vi "LC_Relay_Protection.vi"(0 "Protection settings":T4, 1 "Reset Relay":bool, 3 "RMS minimum\nvalues":cluster{"VRMS values":dbl, "IRMS values":dbl}, 5 "RMS values":dbl[](array[numeric]), 9 "Total power values":dbl[](array[numeric]), 11 "input cluster":T3, 12 "Blocking in":bool, 14 "Transfer Trip":bool) -> (4 "trip signal":bool, 6 "Reclose":bool, 8 "Relay State":cluster{"Lockout":bool, "State":i16}, 10 "Blocking out":bool[](array[boolean]), 13 "millisecond timer value":u32, 15 "output cluster":T3)   [LabVIEW 2016]
doc: "Compares voltage and current RMS values with user defined protection settings to detect undervoltage and overcurrent and calculate trip time.\nImplements definite time and inverse time protection."
uses:
  <vilib>/addons/Electrical Power/Protection/Definite Time Delay/subVIs/fpga_Timer Feedback Var.ctl
  <vilib>/addons/Electrical Power/Protection/Definite Time Delay/subVIs/fpga_State.ctl
  <vilib>/addons/Electrical Power/Protection/Inverse Time Delay/subVIs/ep_Operate Time.ctl
  <vilib>/addons/Electrical Power/Protection/NI_EP_Protection.lvlib
  <vilib>/addons/Electrical Power/Protection/NI_EP_Protection_FPGA.lvlib
panel:
  out "VL error":i32
  out "VR error":i32
  out "I error":i32
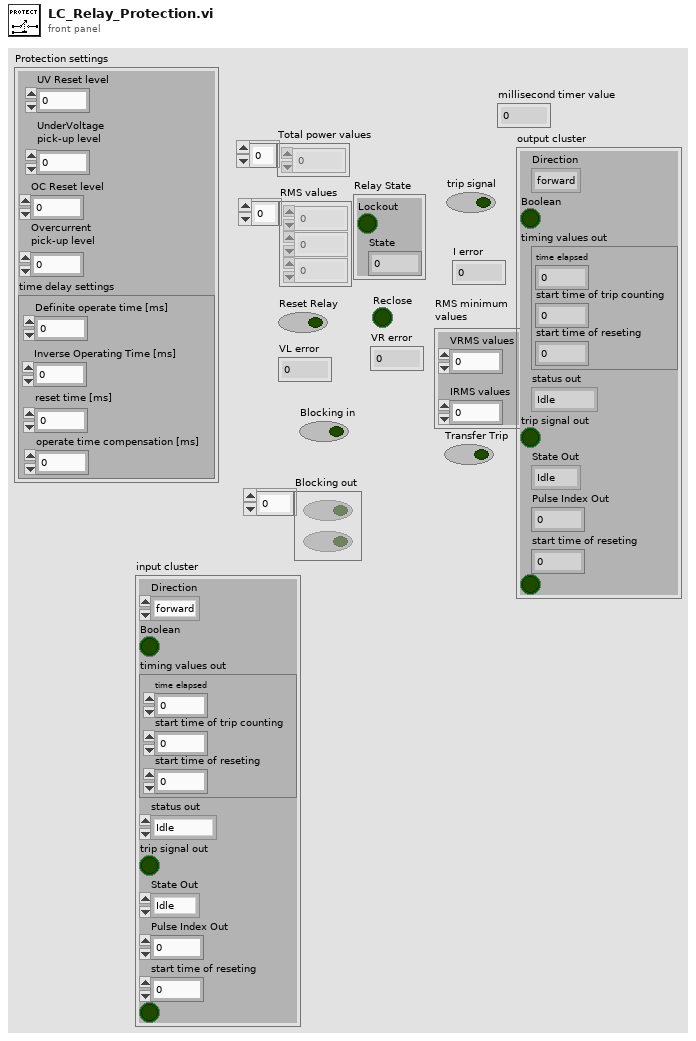
[diagram p1: front panel]
types:
  T1 = typedef "NI_EP_Protection_FPGA.lvlib/fpga_Timer Feedback Var.ctl" = cluster{"time elapsed":u32, "start time of trip counting":u32, "start time of reseting":u32}
  T2 = typedef "NI_EP_Protection_FPGA.lvlib/fpga_State.ctl" = enum16{"Idle", "Trip Counting", "Tripped", "Reset Counting"}
  T3 = cluster{"Direction":enum16{"forward", "backward", "N/D"}, "Boolean":bool, "timing values out":T1, "status out":T2, "trip signal out":bool, "State Out":enum16{"Idle", "Wait for Trip", "PulseClosing", "Locked"}, "Pulse Index Out":i32, "start time of reseting":u32, bool}
  T4 = cluster{"UV Reset level":dbl, "UnderVoltage \npick-up level":dbl, "OC Reset level":dbl, "Overcurrent\npick-up level":dbl, "time delay settings":cluster{"Definite operate time [ms]":u32, "Inverse Operating Time [ms]":u32, "reset time [ms]":u32, "operate time compensation [ms]":u32}}
  T5 = enum16{"Idle", "Wait for Trip", "PulseClosing", "Locked"}
  T6 = cluster{"Definite operate time [ms]":u32, "Inverse Operating Time [ms]":u32, "reset time [ms]":u32, "operate time compensation [ms]":u32}
  T7 = typedef "NI_EP_Protection.lvlib/ep_Operate Time.ctl" = cluster{"A [s]":dbl, "B [s]":dbl, "alpha":dbl, "K2 [s]":dbl, "K1 [s]":dbl, "K3 [s]":dbl}
  T8 = cluster{u32, "reset time [ms]":u32, "reset time [ms]":u32}
  T9 = cluster{"Definite operate time [ms]":u32, "reset time [ms]":u32, "reset time [ms]":u32}
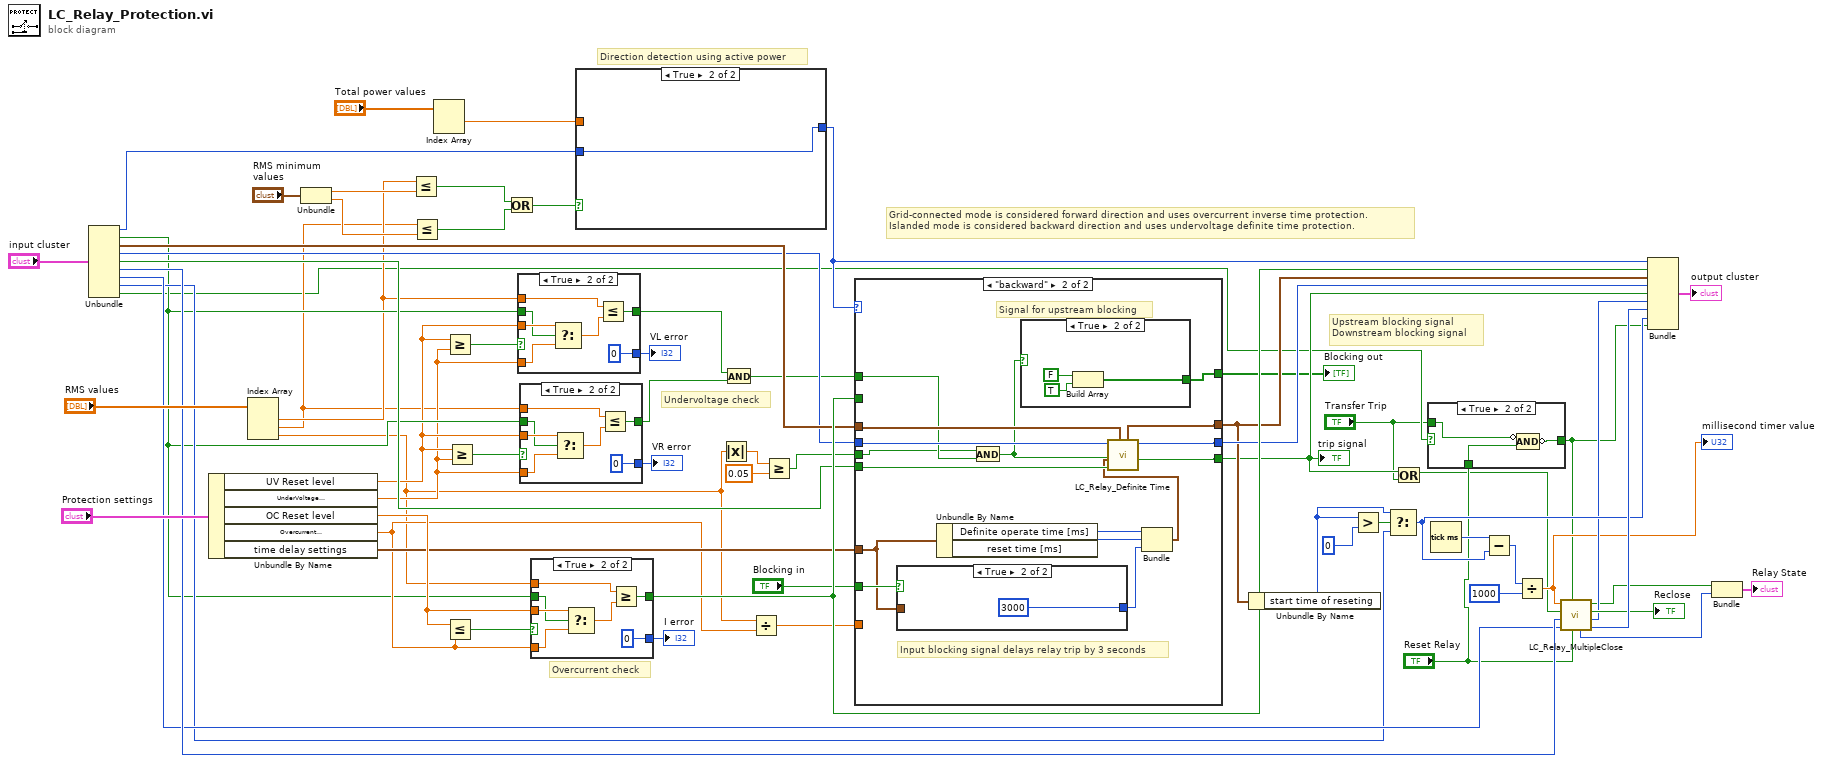
[diagram p0: block diagram]
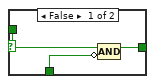
[diagram p2: hidden frame]
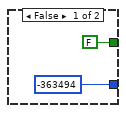
[diagram p3: hidden frame]
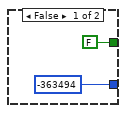
[diagram p4: hidden frame]
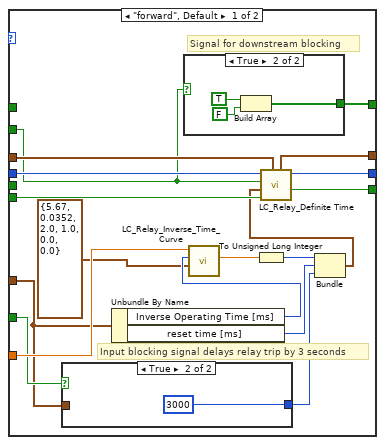
[diagram p5: hidden frame]
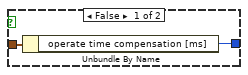
[diagram p6: hidden frame]
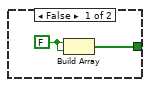
[diagram p7: hidden frame]
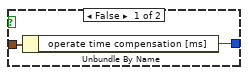
[diagram p8: hidden frame]
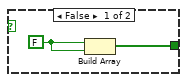
[diagram p9: hidden frame]
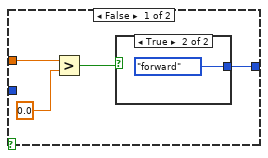
[diagram p10: hidden frame]
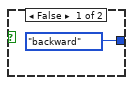
[diagram p11: hidden frame]
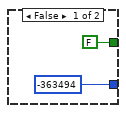
[diagram p12: hidden frame]
diagram:
  # "Grid-connected mode is considered forward direction and uses overcurrent inverse time protection.\nIslanded mode is considered backward direction and uses undervoltage definite time protection."
  # "Overcurrent check"
  # "Undervoltage check"
  # "Direction detection using active power"
  # "Upstream blocking signal\nDownstream blocking signal"
  n1 = Unbundle("input cluster") -> ("Direction"=w44:enum16{"forward", "backward", "N/D"}, "Boolean"=w25:bool, "timing values out"=w31:T1, "status out"=w30:T2, "trip signal out"=w29:bool, "State Out"=w28:T5, "Pulse Index Out"=w27:i32, "start time of reseting"=w26:u32, w7:bool)
  n2 = Unbundle By Name("Protection settings") -> ("UV Reset level"=w24:dbl, "UnderVoltage \npick-up level"=w23:dbl, "OC Reset level"=w59:dbl, "Overcurrent\npick-up level"=w46:dbl, "time delay settings"=w57:T6)
  n3 = Index Array(array="RMS values") -> (element #1=w22:dbl, element #2=w21:dbl, element #3=w18:dbl)  [unwired: 3 in]
  n4 = Unbundle("RMS minimum\nvalues") -> ("VRMS values"=w64:dbl, "IRMS values"=w61:dbl)
  n5 = Less Or Equal?(x=w22, y=w64) -> (x <= y?=w63:bool)
  n6 = Less Or Equal?(x=w21, y=w61) -> (x <= y?=w62:bool)
  n7 = Index Array(array="Total power values") -> (element #1=w50:dbl)  [unwired: 2 in, 1 out]
  n8 = Greater Or Equal?(x=w24, y=w23) -> (x >= y?=w33:bool)
  n9 = Less Or Equal?(x=w59, y=w46) -> (x <= y?=w67:bool)
  n10 = Greater Or Equal?(x=w24, y=w23) -> (x >= y?=w35:bool)
  n11 = Or(x=w63, y=w62) -> (x .or. y?=w54:bool)
  n12 = case shown="True" w33 {
    tunnel: [-363494 ("error") 0 ("error")] -> w32
    tunnel: w24 -> [_ w74]
    tunnel: w23 -> [_ w73]
    tunnel: [FALSE ("Boolean") w72] -> w20
    tunnel: w25 -> [_ w71]
    tunnel: w22 -> [_ w70]
    frame False {
    }
    frame True {
      n13 = Select(t=w74, s=w71, f=w73) -> (s? t:f=w76:dbl)
      n14 = Less Or Equal?(x=w70, y=w76) -> (x <= y?=w72:bool)
    }
  }
  "VL error" <- w32
  n15 = case shown="True" w35 {
    tunnel: [-363494 ("error") 0 ("error")] -> w34
    tunnel: w24 -> [_ w83]
    tunnel: w23 -> [_ w82]
    tunnel: [FALSE ("Boolean") w81] -> w19
    tunnel: w25 -> [_ w80]
    tunnel: w21 -> [_ w79]
    frame False {
    }
    frame True {
      n16 = Select(t=w83, s=w80, f=w82) -> (s? t:f=w85:dbl)
      n17 = Less Or Equal?(x=w79, y=w85) -> (x <= y?=w81:bool)
    }
  }
  "VR error" <- w34
  n18 = case shown="True" w67 {
    tunnel: [-363494 ("error") 0 ("error")] -> w66
    tunnel: w59 -> [_ w92]
    tunnel: w46 -> [_ w91]
    tunnel: [FALSE ("Boolean") w90] -> w58
    tunnel: w25 -> [_ w89]
    tunnel: w18 -> [_ w88]
    frame False {
    }
    frame True {
      n19 = Select(t=w92, s=w89, f=w91) -> (s? t:f=w94:dbl)
      n20 = Greater Or Equal?(x=w88, y=w94) -> (x >= y?=w90:bool)
    }
  }
  "I error" <- w66
  n21 = case shown="True" w54 {
    tunnel: w50 -> [w96 _]
    tunnel: w44 -> [_ w101]
    tunnel: [w95 w101] -> w43
    frame False {
      n22 = Greater?(x=w96, y=0.0) -> (0:w97:bool)
      n23 = case shown="True" w97 {
        tunnel: [enum16{"forward", "backward"}."backward" enum16{"forward", "backward"}."forward"] -> w95
        frame False {
        }
        frame True {
        }
      }
    }
    frame True {
    }
  }
  n24 = Absolute Value(x=w18) -> (abs(x)=w14:dbl)
  n25 = And(x=w20, y=w19) -> (x .and. y?=w16:bool)
  n26 = Divide(x=w18, y=w46) -> (x/y=w55:dbl)
  n27 = Greater Or Equal?(x=w14, y=0.05) -> (x >= y?=w15:bool)
  n28 = case shown="\"backward\"" w43 {
    tunnel: w58 -> [w102 _]
    tunnel: w57 -> [w105 w134]
    tunnel: [w119 w138] -> w56
    tunnel: w55 -> [w118 _]
    tunnel: [w117 w139] -> w53
    tunnel: [w103 w129] -> w47
    tunnel: w31 -> [w116 w142]
    tunnel: w30 -> [w115 w141]
    tunnel: w29 -> [w114 w140]
    tunnel: [w107 w137] -> w37
    tunnel: "Blocking in" -> [w106 w136]
    tunnel: w15 -> [_ w130]
    tunnel: w16 -> [_ w131]
    frame "forward", Default {
      # "Input blocking signal delays relay trip by 3 seconds"
      # "Signal for downstream blocking"
      n29 = case shown="True" w106 {
        tunnel: [w120 u32 3000 ("reset time [ms]")] -> w104
        tunnel: w105 -> [w121 _]
        frame False {
          n30 = Unbundle By Name(w121) -> ("operate time compensation [ms]"=w120:u32)
        }
        frame True {
        }
      }
      n31 = Unbundle By Name(w105) -> ("Inverse Operating Time [ms]"=w113:u32, "reset time [ms]"=w110:u32)
      n32 = case shown="True" w102 {
        tunnel: [w123 w125] -> w107
        frame False {
          w124 = FALSE
          n33 = Build Array(w124, w124) -> (w123:bool[])
        }
        frame True {
          n34 = Build Array(TRUE, FALSE) -> (w125:bool[])
        }
      }
      n35 = call "LC_Relay_Inverse_Time_Curve.vi"("input cluster"=T7 {"A [s]"=5.67, "B [s]"=0.0352, "alpha"=2.0, "K2 [s]"=1.0, "K1 [s]"=0.0, "K3 [s]"=0.0}, "time dial"=w113, "multiples of pickup"=w118) -> ("oparate time"=w111:dbl)  [unwired: 5 in, 1 out]
      n36 = To Unsigned Long Integer(number=w111) -> (unsigned 32bit integer=w108:u32)
      n37 = Bundle(w108, "reset time [ms]"=w110, "reset time [ms]"=w104) -> (w109:T8)  [unwired: 1 in]
      n38 = call "LC_Relay_Definite Time.vi"("timing values in"=w116, "trip signal in"=w114, "time delay settings"=w109, "pick-up signal? (F)"=w102, "status in"=w115) -> ("trip signal out"=w103:bool, "status out"=w119:T2, "timing values out"=w117:T1)  [unwired: 3 in, 1 out]
    }
    frame "backward" {
      # "Signal for upstream blocking"
      # "Input blocking signal delays relay trip by 3 seconds"
      n39 = case shown="True" w136 {
        tunnel: [w144 u32 3000 ("reset time [ms]")] -> w135
        tunnel: w134 -> [w145 _]
        frame False {
          n40 = Unbundle By Name(w145) -> ("operate time compensation [ms]"=w144:u32)
        }
        frame True {
        }
      }
      n41 = Unbundle By Name(w134) -> ("Definite operate time [ms]"=w133:u32, "reset time [ms]"=w143:u32)
      n42 = And(x=w130, y=w131) -> (x .and. y?=w128:bool)
      n43 = case shown="True" w128 {
        tunnel: [w147 w149] -> w137
        frame False {
          w148 = FALSE
          n44 = Build Array(w148, w148) -> (w147:bool[])
        }
        frame True {
          n45 = Build Array(FALSE, TRUE) -> (w149:bool[])
        }
      }
      n46 = Bundle("Definite operate time [ms]"=w133, "reset time [ms]"=w143, "reset time [ms]"=w135) -> (w132:T9)  [unwired: 1 in]
      n47 = call "LC_Relay_Definite Time.vi"("timing values in"=w142, "trip signal in"=w140, "time delay settings"=w132, "pick-up signal? (F)"=w128, "status in"=w141) -> ("trip signal out"=w129:bool, "status out"=w138:T2, "timing values out"=w139:T1)  [unwired: 3 in, 1 out]
    }
  }
  "trip signal" <- w47
  "Blocking out" <- w37
  n48 = Unbundle By Name(w53) -> ("start time of reseting"=w40:u32)
  n49 = Greater?(x=w40, y=u32 0 ("x")) -> (0:w41:bool)
  n50 = Select(t=w40, s=w41, f=w26) -> (s? t:f=w39:u32)
  n51 = Or(x=w47, y="Transfer Trip") -> (x .or. y?=w2:bool)
  n52 = case shown="True" w7 {
    tunnel: "Reset Relay" -> [w153 w156]
    tunnel: [w154 w157] -> w6
    tunnel: "Transfer Trip" -> [w152 w155]
    frame False {
      n53 = Compound Arithmetic op=AND(w152, invert w153) -> (w154:bool)
    }
    frame True {
      n54 = Compound Arithmetic op=AND(invert w155, w156) -> (invert w157:bool)
    }
  }
  n55 = Tick Count (ms)() -> (millisecond timer value=w12:u32)
  n56 = Subtract(x=w12, y=w39) -> (x-y=w13:u32)
  n57 = Divide(x=w13, y=u32 1000) -> (x/y=w11:dbl)
  "millisecond timer value" <- w11
  n58 = call "LC_Relay_MultipleClose.vi"("Reset Relay"="Reset Relay", "Transfer Trip"=w6, "Pulse Index In"=w27, "State In"=w28, "Trip signal"=w2, "Time lapsed"=w11) -> ("Pulse Index Out"=w48:i32, "State Out"=w38:T5, "Reclose"=→"Reclose":bool, "Lockout"=w5:bool, "State"=w4:i16)  [unwired: 1 in]
  n59 = Bundle("Direction"=w43, "Boolean"=w58, "timing values out"=w53, "status out"=w56, "trip signal out"=w47, "State Out"=w38, "Pulse Index Out"=w48, "start time of reseting"=w39, w6) -> (→"output cluster":T3)  [unwired: 1 in]
  n60 = Bundle("Lockout"=w5, "State"=w4) -> (→"Relay State":cluster{"Lockout":bool, "State":i16})  [unwired: 1 in]
